vi "Read ADCs in Engineering Units.vi"(11 "ILC in":refnum<class "ILC.lvclass">) -> (2 "ADCs in Engineering Units":T1 {"Ch5" format="%.1f"; "Ch4" format="%.1f"; "Ch3" format="%.1f"; "Ch2" format="%.1f"; "Ch1" format="%.1f"}, 3 "ILC out":refnum<class "ILC.lvclass">)   [LabVIEW 2013, in "ILCCommon.lvlib" / "ILC.lvclass"]
uses:
  <userlib>/Common/ILC/ILC/ILC.lvclass
  <userlib>/Common/ILC/Typedefs/ADCsInEngineeringUnits.ctl
  <userlib>/Common/ILC/ILC/ILC.lvclass/ILC.ctl
  <userlib>/Common/ILC/Typedefs/ILCTypedefs.lvlib
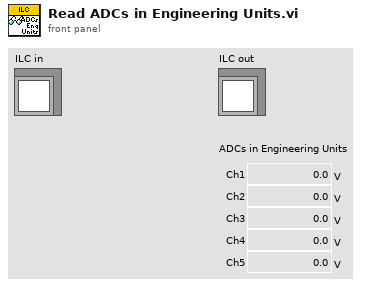
[diagram p1: front panel]
types:
  T1 = typedef "ILCCommon.lvlib/ILCTypedefs.lvlib/ADCsInEngineeringUnits.ctl" = cluster{"Ch1":dbl[unit], "Ch2":dbl[unit], "Ch3":dbl[unit], "Ch4":dbl[unit], "Ch5":dbl[unit]}
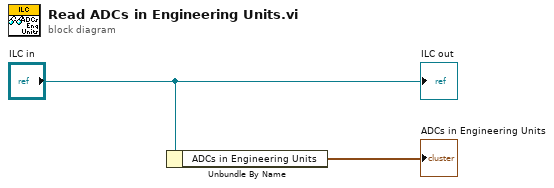
[diagram p0: block diagram]
diagram:
  n1 = Unbundle By Name("ILC in") -> ("ADCs in Engineering Units"=→"ADCs in Engineering Units":T1)
  "ILC out" <- "ILC in"
